vi "Configuration Tool Main.vi"() -> ()   [LabVIEW 2019, in "Configuration Tool.lvlib"]
doc: "This is the main VI for the configuration editor."
uses:
  Configuration Tool.lvlib
  Controls/StateCluster.ctl
  <vilib>/NI/Configuration Framework/Repository/NISE_CEF_Repository.lvclass
  <vilib>/NI/Configuration Framework/Node/NodeRef.ctl
  <vilib>/NI/Configuration Framework/Node/NISE_CEF_Node.lvclass
  <vilib>/NI/Configuration Framework/Node/StandardEvents.ctl
  <vilib>/NI/Configuration Framework/Node/UserEventRef.ctl
  <vilib>/NI/Configuration Framework/Controls/EventCluster.ctl
  <vilib>/NI/Configuration Framework/Node/NodeChangeEvent.ctl
  <vilib>/NI/Configuration Framework/Node/CacheState.ctl
  <vilib>/NI/Configuration Framework/Node/RefreshUIEvent.ctl
  <vilib>/NI/Configuration Framework/Node/StopEvent.ctl
  <vilib>/NI/Configuration Framework/glyph manager/glyph manager.ctl
  <vilib>/picture/picture.llb/imagedata.ctl
  Controls/AddMessage.ctl
  Controls/MoveMessage.ctl
  <vilib>/Utility/error.llb/DialogType.ctl
  Classes/CustomDeviceRepo/CustomDeviceRepo.lvclass
  C:/Program Files (x86)/National Instruments/LabVIEW 2019/vi.lib/NI/Configuration Framework/Repository/NISE_CEF_Repository.lvclass
  <vilib>/Utility/sysdir.llb/System Directory Type.ctl
  <vilib>/NI/AMC/Read Termination Message.vi
  <vilib>/NI/AMC/Create Single Message.vi
  <vilib>/NI/AMC/Update Message Routing Info.vi
  subVI/Global Settings.vi
  <vilib>/NI/AMC/Globals.vi
  <vilib>/NI/AMC/Send Message.vi
  <vilib>/NI/AMC/AMC.lvlib
  <vilib>/NI/Configuration Framework/NISE_CEF_TreeControl.lvlib
  <vilib>/NI/Configuration Framework/glyph manager/glyph manager.lvlib
panel:
  in  "Target Project":string(combo)
  in  "VeriStand Version":string(combo)
  in  "View":string(tree)
  in  "Exit":bool
  out "Status":string
  # "Custom Device XML Editor"
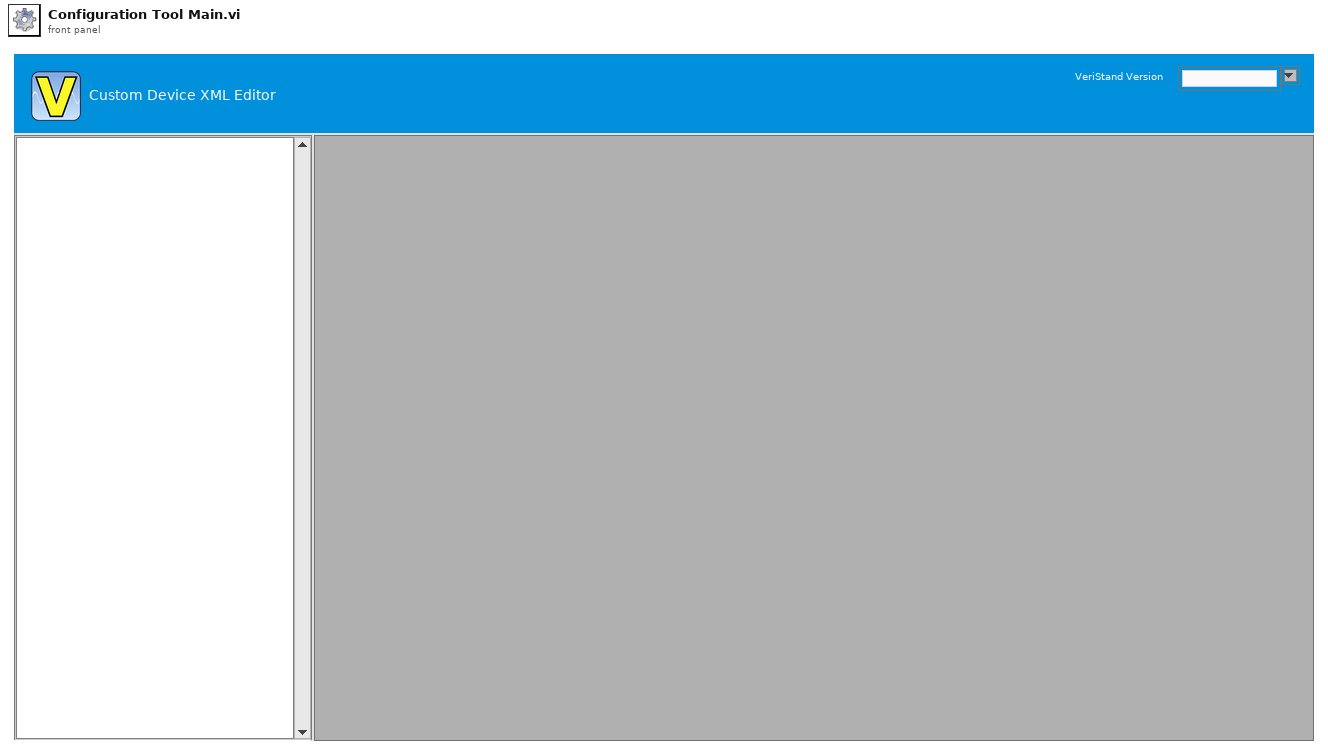
[diagram p1: front panel]
types:
  T1 = typedef "Configuration Tool.lvlib/StateCluster.ctl" = cluster{"repository":refnum<class "NISE_CEF_Repository.lvclass">, "root":T2, "unsaved changes":bool, "current path":path, "standard events":T3, "classes path":path, "glyph manager":T9}
  T2 = typedef "NISE_CEF_Node.lvclass/NodeRef.ctl" = refnum<data-value>
  T3 = typedef "NISE_CEF_Node.lvclass/StandardEvents.ctl" = cluster{"user event":T4, "node change":T5, "cache state":T6, "refresh UI":T7, "stop event":T8}
  T4 = typedef "NISE_CEF_Node.lvclass/UserEventRef.ctl" = refnum<user-event>
  T5 = typedef "NISE_CEF_Node.lvclass/NodeChangeEvent.ctl" = refnum<user-event>
  T6 = typedef "NISE_CEF_Node.lvclass/CacheState.ctl" = refnum<user-event>
  T7 = typedef "NISE_CEF_Node.lvclass/RefreshUIEvent.ctl" = refnum<user-event>
  T8 = typedef "NISE_CEF_Node.lvclass/StopEvent.ctl" = refnum<user-event>
  T9 = typedef "glyph manager.lvlib/glyph manager.ctl" = cluster{"search paths":path[], "glyph map":variant, "base glyphs":T10[], "desired overlays":string[]}
  T10 = typedef "imagedata.ctl" = cluster{"image type":i32, "image depth":i32, "image":u8[], "mask":u8[], "colors":u32[], "Rectangle":cluster{"left":i16, "top":i16, "right":i16, "bottom":i16}}
  T11 = cluster{"Names":string[], "Project refs":refnum<vi>[]}
  T12 = typedef "AMC.lvlib/Message Queue.ctl" = refnum<queue>
  T13 = typedef "Configuration Tool.lvlib/AddMessage.ctl" = cluster{"node type":string, "to add to":string}
  T14 = typedef "Configuration Tool.lvlib/MoveMessage.ctl" = cluster{"node ref":T2, "new parent":T2}
  T15 = typedef "Configuration Tool.lvlib/FilePaths.ctl" = cluster{"glyphs":path, "classes":path}
  T16 = typedef "DialogType.ctl" = u16
  T17 = typedef "System Directory Type.ctl" = i32
  T18 = typedef "NISE_CEF_Node.lvclass/Summary.ctl" = cluster{"ID":string, "parent ID":string, "node type":string, "text":string, "additional text":string, "glyph":string, "depth":i32, "glyph overlay":string}
  T19 = typedef "LVPoint32TypeDef.ctl" = cluster{"Horizontal":i32, "Vertical":i32}
  T20 = cluster{"data name":string, "drag data":variant}[]
  T21 = typedef "NISE_CEF_Node.lvclass/NodeMenuOptions.ctl" = cluster{"removable":bool, "movable":bool, "duplicate":bool}
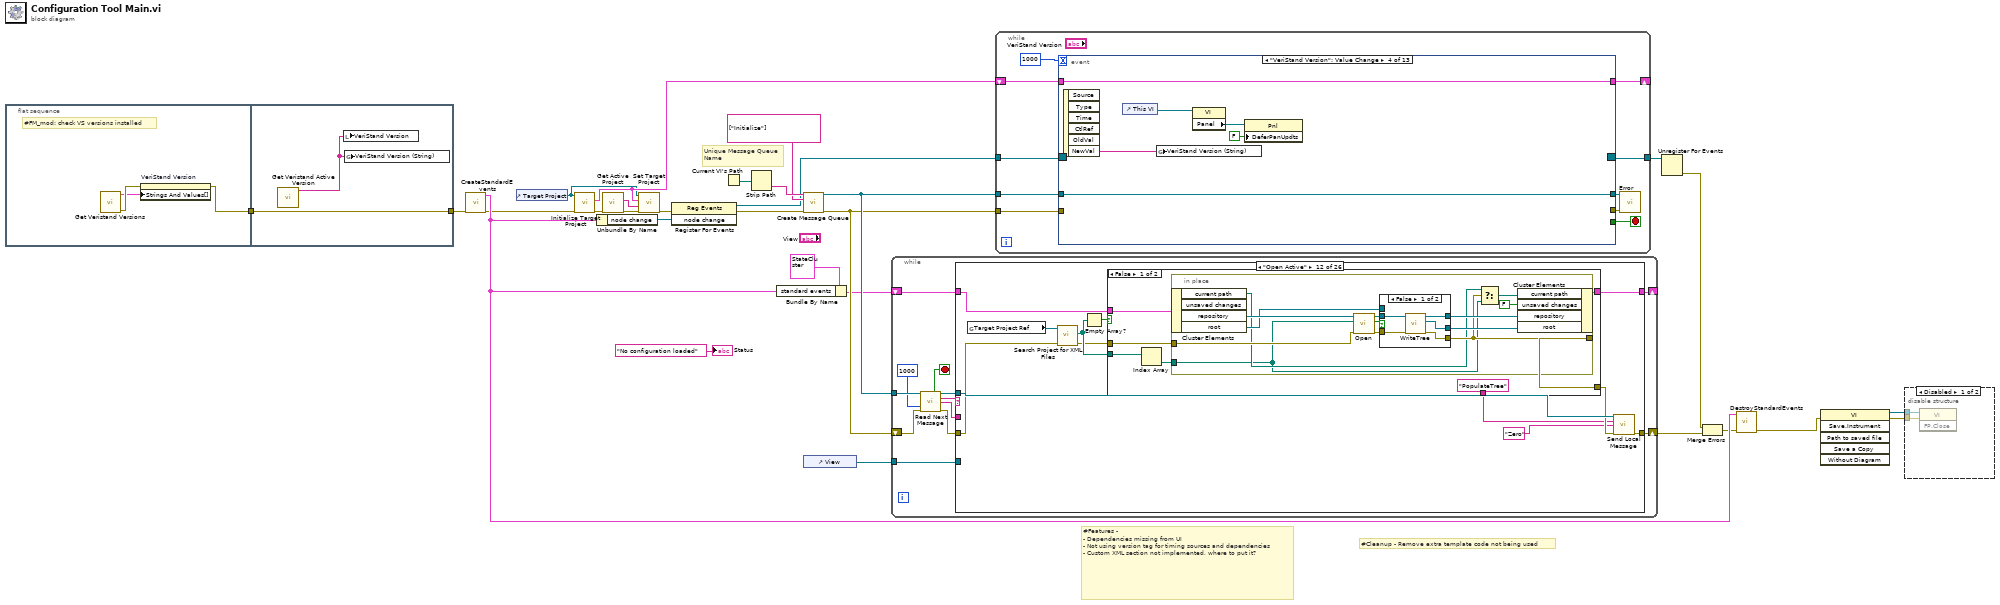
[diagram p0: block diagram]
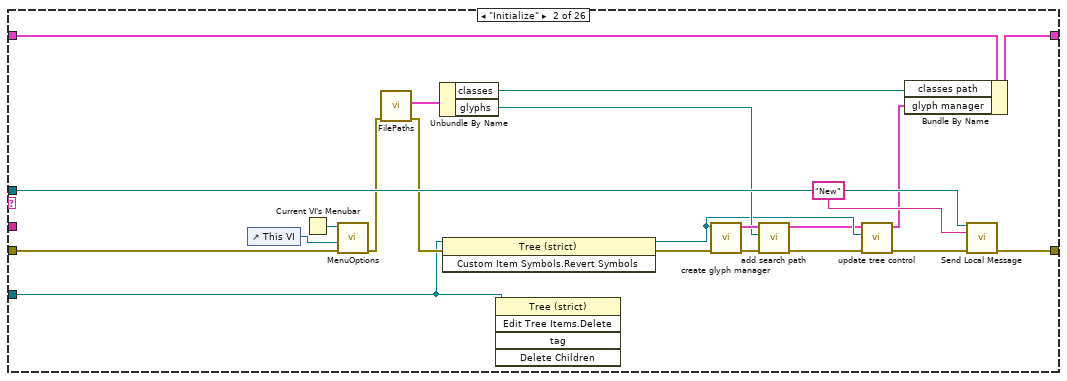
[diagram p4: hidden frame]
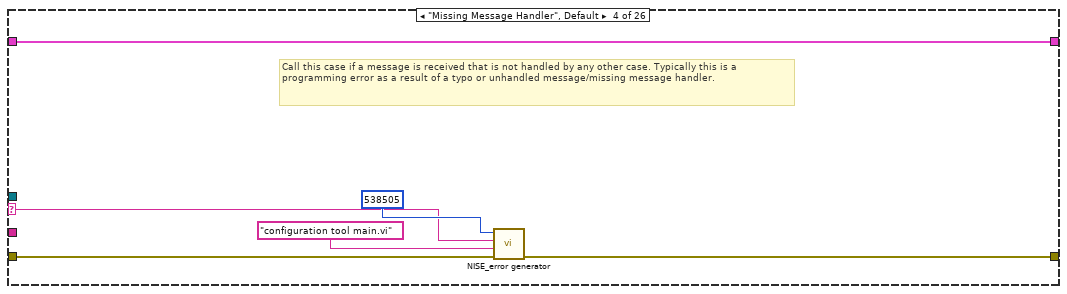
[diagram p6: hidden frame]
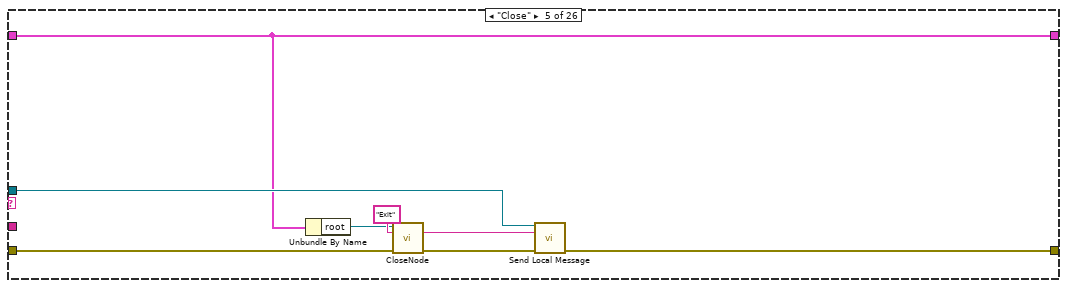
[diagram p7: hidden frame]
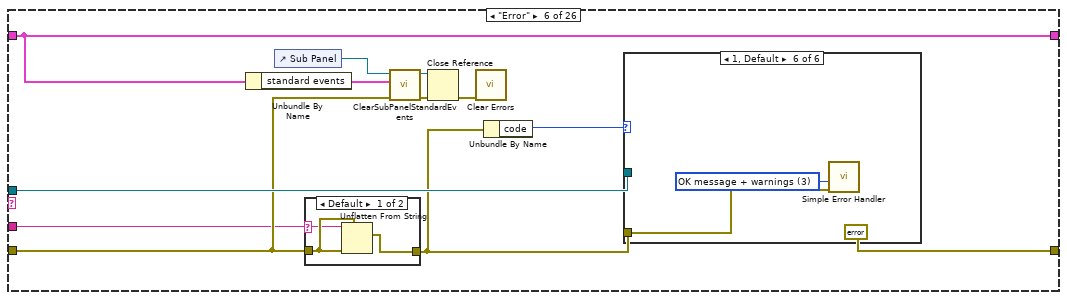
[diagram p8: hidden frame]
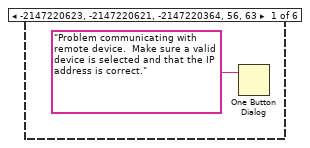
[diagram p10: hidden frame]
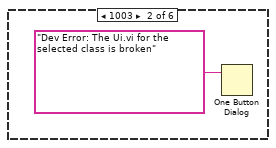
[diagram p11: hidden frame]
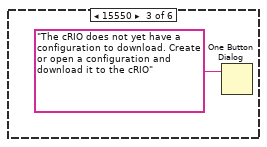
[diagram p12: hidden frame]
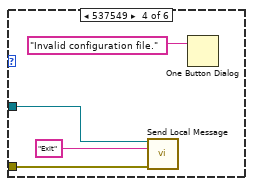
[diagram p13: hidden frame]
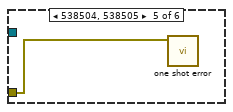
[diagram p14: hidden frame]
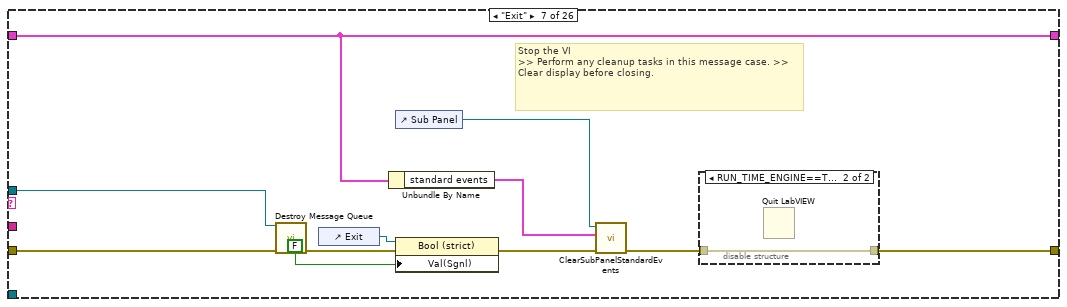
[diagram p15: hidden frame]
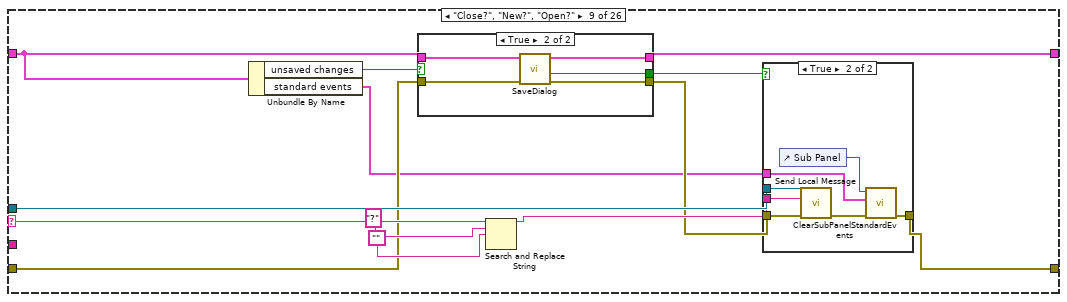
[diagram p18: hidden frame]
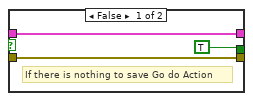
[diagram p19: hidden frame]
diagram:
  # "#Cleanup - Remove extra template code not being used"
  # "#Features - \n- Dependencies missing from UI\n- Not using version tag for timing sources and dependencies\n- Custom XML section not implemented, where to put it?"
  # "Unique Message Queue Name"
  n1 = flat-sequence {
    tunnel: [w31] -> w1
    tunnel: [w34] -> w2
    tunnel: w1 -> [w34]
    frame #0 {
      # "#FM_mod: check VS versions installed"
      n2 = call "Get Veristand Versions.vi"() -> ("error out"=w32:errorcluster, "Versions"=w30:cluster{"String":string, "Value":string}[])  [unwired: 10 in]
      n3 = property on="VeriStand Version" class="CmbBox"(error in=w32, "Strings And Values[]"=w30) -> (error out=w31:errorcluster)  [unwired: 1 in, 1 out]
    }
    frame #1 {
      n4 = call "Get Veristand Active Version.vi"() -> ("Version"=w33:string)  [unwired: 11 in]
      n5 = local write "VeriStand Version"(w33) -> ()
      n6 = global write "Global Settings.vi" "VeriStand Version (String)"(w33) -> ()
    }
  }
  n7 = call <vilib>:"CreateStandardEvents.vi"("error in"=w2) -> ("error out"=w8:errorcluster, "standard events"=w19:T3)  [unwired: 9 in]
  n8 = control-ref of="Target Project"() -> (w9:refnum<vi>)
  n9 = call "Initialize Target Project.vi"("error in (no error)"=w8, "ComboBox in"=w9) -> ("error out"=w13:errorcluster, "Projects"=w11:T11)  [unwired: 8 in]
  n10 = Unbundle By Name(w19) -> ("node change"=w24:T5)
  n11 = call "Get Active Project.vi"("error in (no error)"=w13) -> ("error out"=w12:errorcluster, "Name"=w10:string)  [unwired: 7 in, 2 out]
  n12 = call "Set Target Project.vi"("error in (no error)"=w12, "Target Project"=w10, "Projects"=w11, "ComboBox Ref"=w9) -> ("error out"=w7:errorcluster)  [unwired: 7 in]
  n13 = register-events(error in=w7, w24) -> (reference out=w18:refnum<event-registration>, error out=w23:errorcluster)  [unwired: 1 in]
  n14 = Current VI's Path() -> (path=w28:path)
  n15 = Strip Path(path=w28) -> (name=w29:string)  [unwired: 1 out]
  n16 = Bundle By Name(cluster=T1 {"repository"=refnum, "root"=refnum, "unsaved changes"=FALSE, "current path"=path "", "standard events"={"user event"=refnum, "node change"=refnum, "cache state"=refnum, "refresh UI"=refnum, "stop event"=refnum}, "classes path"=path "", "glyph manager"={"search paths"=[], "glyph map"=variant, "base glyphs"=[], "desired overlays"=[]}}, "standard events"=w19) -> (w21:T1)
  n17 = call <vilib>:"Create Message Queue.vi"("message queue name"=w29, "initial message names"=string[] ["Initialize"], "error in"=w23) -> ("message queue out"=w26:T12, "error out"=w25:errorcluster)  [unwired: 11 in]
  n18 = control-ref of="View"() -> (w17:refnum<vi>)
  n19 = while "Message Processor" {
    shift-right: [w42] -> w20
    shift-left: w25 -> [w41]
    tunnel: w26 -> [w40]
    shift-right: [w38] -> _
    shift-left: w21 -> [w37]
    tunnel: w17 -> [w35]
    stop <- w46 stop-if-true
    n20 = call <vilib>:"Read Next Message.vi"("message queue in"=w40, "timeout (1 ms)"=1000, "error in"=w41) -> ("exit process?"=w46:bool, "message queue out"=w36:T12, "message name"=w45:string, "message value"=w44:string, "error out"=w43:errorcluster)  [unwired: 5 in, 3 out]
    n21 = case shown="\"Open Active\"" w45 {
      selector: w45 -> [_ _ _ w74 _ _ _ _ w135 _ _ _ _ _ _ _ _ _ w393 _ _ _ _ _ _ _]
      tunnel: w44 -> [_ _ _ _ _ w87 _ _ _ _ _ _ _ _ w302 _ w354 w371 w391 w443 w467 w479 _ w528 w548 w555]
      tunnel: w43 -> [w48 w70 w72 w77 w80 w90 w122 w126 w128 w166 w185 w228 w272 w294 w309 w322 w347 w370 w396 w445 w466 w496 w518 w527 w546 w556]
      tunnel: [w48 w66 w72 w75 w84 errorcluster {"status"=FALSE, "code"=0, "source"=""} ("error out") w114 w126 w139 w172 w181 w233 w269 w296 w306 w322 w326 w374 w399 w447 w463 w483 w514 w524 w541 w554] -> w42
      tunnel: [w47 w62 w71 w78 w82 w94 w113 w125 w130 w170 w186 w236 w275 w295 w303 w321 w342 w367 w400 w446 w468 w489 w517 w522 w549 w551] -> w38
      tunnel: w37 -> [w47 w63 w71 w78 w82 w94 w113 w125 w131 w168 w187 w237 w274 w293 w304 w321 w345 w368 w400 w438 w468 w498 w517 w522 w549 w557]
      tunnel: w36 -> [_ w65 _ _ w83 w97 w121 _ w138 w171 w183 w235 _ _ w305 _ w323 _ w394 _ _ _ _ w523 w540 w553]
      tunnel: w35 -> [_ w49 _ _ _ _ _ _ _ _ _ _ _ _ _ _ w343 w363 w388 w440 w461 w485 _ _ _ _]
      frame "------------Generic Operations------------" {
        # "Dummy case to add a seperation in the Case Structure menu"
      }
      frame "Initialize" {
        n22 = control-ref of="This VI"() -> (w69:refnum<vi>)
        n23 = Current VI's Menubar() -> (w68:refnum<k9>)
        n24 = call "MenuOptions.vi"("error in"=w70, "VI ref"=w69, "menu ref in"=w68) -> ("error out"=w61:errorcluster)  [unwired: 7 in, 1 out]
        n25 = call "FilePaths.vi"("error in"=w61) -> ("error out"=w54:errorcluster, "paths"=w64:T15)  [unwired: 9 in]
        n26 = Unbundle By Name(w64) -> ("classes"=w60:path, "glyphs"=w56:path)
        n27 = invoke class="Tree (strict)" method="Custom Item Symbols.Revert Symbols"(reference=w49, error in=w54) -> (reference out=w52:refnum<vi>, error out=w53:errorcluster)  [unwired: 1 in, 1 out]
        n28 = invoke class="Tree (strict)" method="Edit Tree Items.Delete"(reference=w49) -> ()  [unwired: 4 in, 5 out]
        n29 = call <vilib>:"create glyph manager.vi"("error in"=w53, "tree ref (for default symbols)"=w52) -> ("error out"=w59:errorcluster, "glyph manager"=w58:T9)  [unwired: 8 in]
        n30 = call <vilib>:"add search path.vi"("error in"=w59, "search path"=w56, "glyph manager in"=w58) -> ("error out"=w51:errorcluster, "glyph manager out"=w50:T9)  [unwired: 7 in]
        n31 = call <vilib>:"update tree control.vi"("error in"=w51, "tree reference"=w52, "glyph manager in"=w50) -> ("error out"=w57:errorcluster, "glyph manager out"=w55:T9)  [unwired: 7 in]
        n32 = Bundle By Name(cluster=w63, "classes path"=w60, "glyph manager"=w55) -> (w62:T1)
        n33 = call <vilib>:"Send Local Message.vi"("message queue in"=w65, "message name"="New" ("Message Name"), "error in"=w57) -> ("error out"=w66:errorcluster)  [unwired: 10 in, 2 out]
      }
      frame "", "Idle" {
      }
      frame "Missing Message Handler", Default {
        # "Call this case if a message is received that is not handled by any other case. Typically this is a programming error as a result of a typo or unhandled message/missing message handler."
        n34 = call <vilib>:"NISE_error generator.vi"("error in"=w77, "source"="configuration tool main.vi", "append error message"=w74, "error code (0)"=538505) -> ("error out"=w75:errorcluster)  [unwired: 5 in]
      }
      frame "Close" {
        n35 = Unbundle By Name(w82) -> ("root"=w81:T2)
        n36 = call <vilib>:"CloseNode.vi"("error in"=w80, "node ref"=w81) -> ("error out"=w79:errorcluster)  [unwired: 9 in]
        n37 = call <vilib>:"Send Local Message.vi"("message queue in"=w83, "message name"="Exit", "error in"=w79) -> ("error out"=w84:errorcluster)  [unwired: 10 in, 2 out]
      }
      frame "Error" {
        n38 = Unbundle By Name(w94) -> ("standard events"=w86:T3)
        n39 = control-ref of="Sub Panel"() -> (w93:refnum<vi>)
        n40 = case shown="Default" w87 {
          selector: w87 -> [w99 _]
          tunnel: w90 -> [w100 w101]
          tunnel: [w98 w101] -> w89
          frame Default {
            n41 = Unflatten From String(type=w100, binary string=w99, error in (no error)=w100) -> (value=w98:errorcluster)  [unwired: 2 in, 2 out]
          }
          frame "" {
          }
        }
        n42 = call <vilib>:"ClearSubPanelStandardEvents.vi"("error in"=w90, "standard events"=w86, "sub panel ref in"=w93) -> ("error out"=w92:errorcluster, "sub panel ref out"=w91:refnum<vi>)  [unwired: 7 in]
        n43 = Close Reference(reference=w91, error in (no error)=w92) -> (error out=w88:errorcluster)
        n44 = call <vilib>:"Clear Errors.vi"("error in (no error)"=w88) -> ()  [unwired: 5 in, 2 out]
        n45 = Unbundle By Name(w89) -> ("code"=w95:i32)
        n46 = case shown="1, Default" w95 {
          tunnel: w97 -> [_ _ _ w107 _ _]
          tunnel: w89 -> [_ _ _ w106 w109 w111]
          frame -2147220623, -2147220621, -2147220364, 56, 63 {
            n47 = One Button Dialog(message="Problem communicating with remote device.  Make sure a valid device is selected and that the IP address is correct.") -> ()  [unwired: 1 in, 1 out]
          }
          frame 1003 {
            n48 = One Button Dialog(message="Dev Error: The Ui.vi for the selected class is broken") -> ()  [unwired: 1 in, 1 out]
          }
          frame 15550 {
            n49 = One Button Dialog(message="The cRIO does not yet have a configuration to download. Create or open a configuration and download it to the cRIO") -> ()  [unwired: 1 in, 1 out]
          }
          frame 537549 {
            n50 = call <vilib>:"Send Local Message.vi"("message queue in"=w107, "message name"="Exit", "error in"=w106) -> ()  [unwired: 10 in, 3 out]
            n51 = One Button Dialog(message="Invalid configuration file.") -> ()  [unwired: 1 in, 1 out]
          }
          frame 538504, 538505 {
            n52 = call <vilib>:"one shot error.vi"("error in"=w109) -> ()  [unwired: 11 in]
          }
          frame 1, Default {
            w110 = T16 3 items=["no dialog", "OK message", "continue or stop message", "OK message + warnings", "continue/stop + warnings"] ("type of dialog (OK msg:1)")
            n53 = call <vilib>:"Simple Error Handler.vi"("type of dialog (OK msg:1)"=w110, "error in (no error)"=w111) -> ()  [unwired: 8 out]
          }
        }
      }
      frame "Exit" {
        # "Stop the VI                                                                             >> Perform any cleanup tasks in this message case. >> Clear display before closing."
        n54 = call <vilib>:"Destroy Message Queue.vi"("message queue in"=w121, "error in"=w122) -> ("error out"=w118:errorcluster)  [unwired: 11 in, 2 out]
        n55 = control-ref of="Exit"() -> (w120:refnum<vi>)
        n56 = Unbundle By Name(w113) -> ("standard events"=w112:T3)
        n57 = control-ref of="Sub Panel"() -> (w117:refnum<vi>)
        n58 = property class="Bool (strict)"(reference=w120, error in=w118, "Val(Sgnl)"=FALSE ("Exit")) -> (error out=w116:errorcluster)  [unwired: 1 out]
        n59 = call <vilib>:"ClearSubPanelStandardEvents.vi"("error in"=w116, "standard events"=w112, "sub panel ref in"=w117) -> ("error out"=w115:errorcluster)  [unwired: 7 in, 1 out]
        n60 = disable-structure shown="RUN_TIME_ENGINE==True" {
          disable-tunnel: [w123 w124] -> w114
          disable-tunnel: w115 -> [w123 w124]
          frame condition #0 (active) {
          }
          frame condition #1 {
            n61 = Quit LabVIEW() -> ()  [unwired: 1 in]
          }
        }
      }
      frame "------------Menu Operations--------------" {
        # "Dummy case to add a seperation in the Case Structure menu"
      }
      frame "Close?", "New?", "Open?" {
        n62 = Unbundle By Name(w131) -> ("unsaved changes"=w133:bool, "standard events"=w127:T3)
        n63 = case shown="True" w133 {
          tunnel: [TRUE ("SaveFlag") w147] -> w132
          tunnel: w131 -> [w141 w146]
          tunnel: [w141 w145] -> w130
          tunnel: w128 -> [w140 w144]
          tunnel: [w140 w143] -> w129
          frame False {
            # "If there is nothing to save Go do Action"
          }
          frame True {
            n64 = call "SaveDialog.vi"("error in"=w144, "state in"=w146) -> ("error out"=w143:errorcluster, "new"=w147:bool, "state out"=w145:T1)  [unwired: 7 in]
          }
        }
        n65 = Search and Replace String(input string=w135, search string="?", replace string="") -> (result string=w134:string)  [unwired: 5 in, 3 out]
        n66 = case shown="True" w132 {
          tunnel: w129 -> [w148 w155]
          tunnel: [w148 w151] -> w139
          tunnel: w138 -> [_ w154]
          tunnel: w134 -> [_ w153]
          tunnel: w127 -> [_ w149]
          frame False {
          }
          frame True {
            n67 = control-ref of="Sub Panel"() -> (w150:refnum<vi>)
            n68 = call <vilib>:"Send Local Message.vi"("message queue in"=w154, "message name"=w153, "error in"=w155) -> ("error out"=w152:errorcluster)  [unwired: 10 in, 2 out]
            n69 = call <vilib>:"ClearSubPanelStandardEvents.vi"("error in"=w152, "standard events"=w149, "sub panel ref in"=w150) -> ("error out"=w151:errorcluster)  [unwired: 7 in, 1 out]
          }
        }
      }
      frame "New" {
        # "#Change - Won't allow creating so changing unsaved constant to F"
        n70 = Unbundle By Name(w168) -> ("classes path"=w167:path)
        n71 = Current VI's Menubar() -> (w162:refnum<k9>)
        n72 = call-dynamic "Initialize.vi"("error in"=w166, "path"=w167, "repository in"=refnum<class "CustomDeviceRepo.lvclass"> refnum ("CustomDeviceRepo.lvclass")) -> ("error out"=w165:errorcluster, "repository out"=w164:refnum<class "CustomDeviceRepo.lvclass">)  [unwired: 7 in]
        n73 = call-dynamic "GenerateMenu.vi"("error in"=w165, "menu ref in"=w162, "NISE_CEF_Repository in"=w164) -> ("error out"=w161:errorcluster, "NISE_CEF_Repository out"=w163:refnum<class "CustomDeviceRepo.lvclass">)  [unwired: 6 in, 1 out]
        n74 = call "Get Active Project.vi"() -> ("No Active Project?"=w159:bool)  [unwired: 8 in, 3 out]
        n75 = Bundle By Name(cluster=w168, "unsaved changes"=FALSE ("SaveFlag"), "repository"=w163) -> (w170:T1)
        n76 = Select(t="Idle", s=w159, f="Open Active") -> (s? t:f=w156:string)
        n77 = call <vilib>:"Send Local Message.vi"("message queue in"=w171, "message name"=w156, "error in"=w161) -> ("error out"=w172:errorcluster)  [unwired: 10 in, 2 out]
      }
      frame "Open" {
        w180 = T17 6 items=["User Home"=0, "User Desktop"=1, "User Documents"=2, "User Application Data"=3, "User Preferences"=4, "User Temporary"=5, "Public Documents"=6, "Public Application Data"=7, "Public Preferences"=8, "Public Cache"=13, "System Core Libraries"=9, "System Installed Libraries"=10, "Application Files"=11, "Boot Volume Root"=12] ("system directory type")
        n78 = disable-structure shown="Disabled" {
          disable-tunnel: [w188 w190] -> w173
          frame Disabled {
            n79 = global read "Global Settings.vi" "VeriStand Version"() -> (w189:enum16{"2013", "2014", "2015", "2016"})
            n80 = Format Into String(w189) -> (resulting string=w188:string)  [unwired: 3 in, 1 out]
          }
          frame Enabled {
            # "#FM_mod: using string instead"
            n81 = global read "Global Settings.vi" "VeriStand Version (String)"() -> (w190:string)
          }
        }
        n82 = Search and Replace String(input string="National Instruments\\NI VeriStand XXXX\\Custom Devices", search string="XXXX", replace string=w173) -> (result string=w176:string)  [unwired: 5 in, 3 out]
        n83 = call <vilib>:"Get System Directory.vi"("system directory type"=w180) -> ("system directory"=w177:path)  [unwired: 10 in]
        n84 = Build Path(base path=w177, name or relative path=w176) -> (appended path=w175:path)
        n85 = in-place {
          in-place-border: w185 -> [w196]
          in-place-border: [w195] -> w182
          in-place-border: w175 -> [w191]
          n86 = in-place-cluster #1(w187) -> ("current path"=w193:path, "repository"=w204:refnum<class "NISE_CEF_Repository.lvclass">, "root"=w200:T2)  [unwired: 1 out]
          n87 = call "FileDialog.vi"("error in"=w196, "start path"=w191) -> ("error out"=w197:errorcluster, "cancelled"=w198:bool, "selected path"=w194:path)  [unwired: 7 in]
          n88 = Compound Arithmetic op=OR(invert w198) -> (w199:bool)
          n89 = case shown="True" w199 {
            tunnel: w204 -> [w205 w217]
            tunnel: [w205 w215] -> w202
            tunnel: [w206 w213] -> w195
            tunnel: [w207 w212] -> w201
            tunnel: w194 -> [_ w210]
            tunnel: w197 -> [w206 w209]
            tunnel: w200 -> [w207 w208]
            frame False {
            }
            frame True {
              n90 = call-dynamic "Open.vi"("error in"=w209, "file path"=w210, "repository in"=w217) -> ("error out"=w214:errorcluster, "invalid?"=w211:bool, "repository out"=w216:refnum<class "NISE_CEF_Repository.lvclass">)  [unwired: 6 in]
              n91 = case shown="False" w211 {
                tunnel: w216 -> [w222 w225]
                tunnel: [w221 w225] -> w215
                tunnel: w214 -> [w220 w224]
                tunnel: [w219 w224] -> w213
                tunnel: [w218 w223] -> w212
                tunnel: w208 -> [_ w223]
                frame False {
                  n92 = call-dynamic "WriteTree.vi"("error in"=w220, "repository in"=w222) -> ("error out"=w219:errorcluster, "root"=w218:T2, "repository out"=w221:refnum<class "NISE_CEF_Repository.lvclass">)  [unwired: 7 in]
                }
                frame True {
                }
              }
            }
          }
          n93 = Select(t=w193, s=w195, f=w194) -> (s? t:f=w192:path)
          n94 = in-place-cluster #1("current path"=w192, "unsaved changes"=FALSE ("SaveFlag"), "repository"=w202, "root"=w201) -> (w186:T1)
        }
        n95 = call <vilib>:"Send Local Message.vi"("message queue in"=w183, "message name"="PopulateTree", "message value"="Zero", "error in"=w182) -> ("error out"=w181:errorcluster)  [unwired: 9 in, 2 out]
      }
      frame "Open Active" {
        n96 = global read "Global Settings.vi" "Target Project Ref"() -> (w231:refnum<vi>)
        n97 = call "Search Project for XML Files.vi"("error in (no error)"=w228, "project reference"=w231) -> ("error out"=w227:errorcluster, "xml files found"=w230:path[])  [unwired: 8 in]
        n98 = Empty Array?(array=w230) -> (empty?=w229:bool)
        n99 = case shown="False" w229 {
          tunnel: w237 -> [w244 w268]
          tunnel: [w243 w268] -> w236
          tunnel: w227 -> [w242 w267]
          tunnel: [w241 w267] -> w234
          tunnel: w230 -> [w239 _]
          tunnel: ["PopulateTree" "Idle"] -> w226
          frame False {
            n100 = Index Array(array=w239) -> (element=w240:path)  [unwired: 1 in]
            n101 = in-place {
              in-place-border: w242 -> [w252]
              in-place-border: [w251] -> w241
              in-place-border: w240 -> [w245]
              n102 = in-place-cluster #2(w244) -> ("current path"=w250:path, "repository"=w257:refnum<class "NISE_CEF_Repository.lvclass">, "root"=w253:T2)  [unwired: 1 out]
              n103 = call-dynamic "Open.vi"("error in"=w252, "file path"=w245, "repository in"=w257) -> ("error out"=w247:errorcluster, "invalid?"=w246:bool, "repository out"=w248:refnum<class "NISE_CEF_Repository.lvclass">)  [unwired: 6 in]
              n104 = case shown="False" w246 {
                tunnel: w248 -> [w262 w265]
                tunnel: [w261 w265] -> w255
                tunnel: w247 -> [w260 w264]
                tunnel: [w259 w264] -> w251
                tunnel: [w258 w263] -> w254
                tunnel: w253 -> [_ w263]
                frame False {
                  n105 = call-dynamic "WriteTree.vi"("error in"=w260, "repository in"=w262) -> ("error out"=w259:errorcluster, "root"=w258:T2, "repository out"=w261:refnum<class "NISE_CEF_Repository.lvclass">)  [unwired: 7 in]
                }
                frame True {
                }
              }
              n106 = Select(t=w250, s=w251, f=w245) -> (s? t:f=w249:path)
              n107 = in-place-cluster #2("current path"=w249, "unsaved changes"=FALSE ("SaveFlag"), "repository"=w255, "root"=w254) -> (w243:T1)
            }
          }
          frame True {
          }
        }
        n108 = call <vilib>:"Send Local Message.vi"("message queue in"=w235, "message name"=w226, "message value"="Zero", "error in"=w234) -> ("error out"=w233:errorcluster)  [unwired: 9 in, 2 out]
      }
      frame "Save" {
        n109 = in-place {
          in-place-border: w272 -> [w279]
          in-place-border: [w278] -> w271
          in-place-border: [w276] -> w270
          n110 = in-place-cluster #3(w274) -> ("current path"=w277:path, "root"=w280:T2, "repository"=w282:refnum<class "NISE_CEF_Repository.lvclass">)
          n111 = Empty String/Path?(string/path=w277) -> (empty?=w276:bool)
          n112 = call-dynamic "ReadTree.vi"("error in"=w279, "root"=w280, "repository in"=w282) -> ("error out"=w278:errorcluster, "repository out"=w281:refnum<class "NISE_CEF_Repository.lvclass">)  [unwired: 7 in]
          n113 = in-place-cluster #3("current path"=w277, "root"=w280, "repository"=w281) -> (w273:T1)
        }
        n114 = case shown="False" w270 {
          tunnel: w273 -> [w286 w288]
          tunnel: [w285 w287] -> w275
          tunnel: [w284 w289] -> w269
          tunnel: w271 -> [w283 w290]
          frame False {
            n115 = call "Save.vi"("error in"=w283, "state in"=w286) -> ("error out"=w284:errorcluster, "state out"=w285:T1)  [unwired: 8 in]
          }
          frame True {
            # "Empty path use Dialog"
            n116 = call "SaveAs.vi"("error in"=w290, "state in"=w288) -> ("error out"=w289:errorcluster, "state out"=w287:T1)  [unwired: 7 in, 1 out]
          }
        }
      }
      frame "SaveAs" {
        n117 = in-place {
          in-place-border: w294 -> [w298]
          in-place-border: [w297] -> w292
          n118 = in-place-cluster #4(w293) -> ("root"=w299:T2, "repository"=w301:refnum<class "NISE_CEF_Repository.lvclass">)
          n119 = call-dynamic "ReadTree.vi"("error in"=w298, "root"=w299, "repository in"=w301) -> ("error out"=w297:errorcluster, "repository out"=w300:refnum<class "NISE_CEF_Repository.lvclass">)  [unwired: 7 in]
          n120 = in-place-cluster #4("root"=w299, "repository"=w300) -> (w291:T1)
        }
        n121 = call "SaveAs.vi"("error in"=w292, "state in"=w291) -> ("error out"=w296:errorcluster, "state out"=w295:T1)  [unwired: 7 in, 1 out]
      }
      frame "Custom View" {
        n122 = in-place {
          in-place-border: w309 -> [w320]
          in-place-border: [w319] -> w307
          in-place-border: w302 -> [w310]
          n123 = in-place-cluster #5(w304) -> ("repository"=w314:refnum<class "NISE_CEF_Repository.lvclass">, "root"=w313:T2)
          n124 = call-dynamic "ReadTree.vi"("error in"=w320, "root"=w313, "repository in"=w314) -> ("error out"=w317:errorcluster, "repository out"=w316:refnum<class "NISE_CEF_Repository.lvclass">)  [unwired: 7 in]
          n125 = call-dynamic "CustomView.vi"("error in"=w317, "view name"=w310, "repository in"=w316) -> ("error out"=w318:errorcluster, "repository out"=w315:refnum<class "NISE_CEF_Repository.lvclass">)  [unwired: 7 in]
          n126 = call-dynamic "WriteTree.vi"("error in"=w318, "repository in"=w315) -> ("error out"=w319:errorcluster, "root"=w311:T2, "repository out"=w312:refnum<class "NISE_CEF_Repository.lvclass">)  [unwired: 7 in]
          n127 = in-place-cluster #5("repository"=w312, "root"=w311) -> (w303:T1)
        }
        n128 = call <vilib>:"Send Local Message.vi"("message queue in"=w305, "message name"="PopulateTree", "error in"=w307) -> ("error out"=w306:errorcluster)  [unwired: 10 in, 2 out]
      }
      frame "-------TreeControl Operations-----------" {
        # "Dummy case to add a seperation in the Case Structure menu"
      }
      frame "AddNode" {
        # "#Change - Added ability for added nodes\nto then add children"
        # "#Change - Had to make own copy\nof add node since CEF framework\ndoesn't let you pass params to init"
        # "#Change - Look for potential\ndashes for menu items with\nparameterized options"
        n129 = Unflatten From String(type=T13 {"node type"="", "to add to"=""} ("input cluster"), binary string=w354) -> (value=w352:T13)  [unwired: 3 in, 2 out]
        n130 = Unbundle By Name(w352) -> ("to add to"=w350:string, "node type"=w332:string)
        n131 = Match Pattern(string=w332, regular expression="\\-") -> (before substring=w331:string, after substring=w330:string)  [unwired: 1 in, 2 out]
        n132 = in-place {
          in-place-border: w347 -> [w360]
          in-place-border: [w359] -> w346
          in-place-border: w331 -> [w358]
          in-place-border: [w357] -> w344
          n133 = in-place-cluster #6(w345) -> ("repository"=w362:refnum<class "NISE_CEF_Repository.lvclass">)
          n134 = call-dynamic "GetClassPath.vi"("error in"=w360, "class name"=w358, "Repository in"=w362) -> ("error out"=w359:errorcluster, "class path"=w357:path, "Repository out"=w361:refnum<class "NISE_CEF_Repository.lvclass">)  [unwired: 6 in]
          n135 = in-place-cluster #6("repository"=w361) -> (w339:T1)
        }
        n136 = Unbundle By Name(w339) -> ("glyph manager"=w338:T9)
        n137 = call <vilib>:"Get LV Class Default Value.vi"("error in (no error)"=w346, "class path"=w344) -> ("error out"=w355:errorcluster, "object"=w356:refnum<class>)  [unwired: 8 in]
        n138 = To More Specific Class(target class=refnum<class "NISE_CEF_Node.lvclass"> refnum ("Node.lvclass"), reference=w356, error in=w355) -> (specific class reference=w340:refnum<class "NISE_CEF_Node.lvclass">, error out=w341:errorcluster)
        n139 = call-dynamic "AddGlyphtoGManager.vi"("error in"=w341, "glyph manager"=w338, "NISE_CEF_Node in"=w340) -> ("error out"=w336:errorcluster, "glyph manager out"=w337:T9, "NISE_CEF_Node out"=w335:refnum<class "NISE_CEF_Node.lvclass">)  [unwired: 6 in]
        n140 = Match Pattern(string=w330, regular expression="\\-") -> (before substring=w328:string, after substring=w325:string)  [unwired: 1 in, 2 out]
        n141 = call "Modified Framework AddNode.vi"("parameters"=w328, "error in"=w336, "node in"=w335, "parent node ID"=w350) -> ("error out"=w349:errorcluster, "summary"=w348:T18[], "ID of Added Node"=w324:string)  [unwired: 5 in]
        n142 = call <vilib>:"PopulateTreeSumaryWithGlyphManager.vi"("error in"=w349, "glyph manager"=w337, "summary"=w348, "tree ref in"=w343) -> ("error out"=w327:errorcluster, "glyph manager out"=w334:T9)  [unwired: 6 in]
        n143 = Bundle By Name(cluster=w339, "glyph manager"=w334) -> (w342:T1)
        n144 = call "Send Message to Create Child Object.vi"("Error In"=w327, "ID of Node to Add To"=w324, "node type"=w325, "Queue in"=w323) -> ("Error Out"=w326:errorcluster)  [unwired: 6 in, 1 out]
      }
      frame "Duplicate" {
        n145 = call <vilib>:"IDtoNode.vi"("error in"=w370, "ID"=w371) -> ("error out"=w372:errorcluster, "invalid Id"=w369:bool, "node ref"=w373:T2)  [unwired: 7 in]
        n146 = Unbundle By Name(w368) -> ("glyph manager"=w365:T9)
        n147 = case shown="False" w369 {
          tunnel: [w385 w387] -> w374
          tunnel: w373 -> [w384 _]
          tunnel: w372 -> [w381 w387]
          tunnel: w365 -> [w377 w386]
          tunnel: [w376 w386] -> w364
          tunnel: w363 -> [w375 _]
          frame False {
            n148 = call <vilib>:"DuplicateNode.vi"("same parent?"=TRUE ("s"), "error in"=w381, "node ref in"=w384) -> ("error out"=w382:errorcluster, "new node ref"=w383:T2)  [unwired: 7 in]
            n149 = call <vilib>:"Summary.vi"("error in"=w382, "node self ref"=w383) -> ("error out"=w379:errorcluster, "summary"=w378:T18[])  [unwired: 8 in]
            n150 = call <vilib>:"PopulateTreeSumaryWithGlyphManager.vi"("error in"=w379, "glyph manager"=w377, "summary"=w378, "tree ref in"=w375) -> ("error out"=w385:errorcluster, "glyph manager out"=w376:T9)  [unwired: 6 in]
          }
          frame True {
          }
        }
        n151 = Bundle By Name(cluster=w368, "unsaved changes"=TRUE, "glyph manager"=w364) -> (w367:T1)
      }
      frame "CustomMenuAction" {
        n152 = Match Pattern(string=w391, regular expression=":") -> (before substring=w390:string, after substring=w389:string)  [unwired: 1 in, 2 out]
        n153 = call <vilib>:"IDtoNode.vi"("error in"=w396, "ID"=w389) -> ("error out"=w397:errorcluster, "invalid Id"=w395:bool, "node ref"=w398:T2)  [unwired: 7 in]
        n154 = case shown="False" w395 {
          tunnel: [w406 w436] -> w399
          tunnel: w398 -> [w403 _]
          tunnel: w397 -> [w409 w436]
          tunnel: w394 -> [w410 _]
          tunnel: w393 -> [_ _]
          tunnel: w390 -> [w407 _]
          tunnel: w388 -> [w404 _]
          frame False {
            n155 = in-place {
              in-place-border: w410 -> [w434]
              in-place-border: w409 -> [w432]
              in-place-border: [w431] -> w405
              in-place-border: [w430] -> w408
              in-place-border: w407 -> [w429]
              in-place-border: w404 -> [w428]
              in-place-border: [w427] -> w402
              n156 = in-place-dvr #7(w403) -> (w435:refnum<class "NISE_CEF_Node.lvclass">)  [unwired: 1 out]
              n157 = call-dynamic "MenuHandler.vi"("tree control"=w428, "main message queue"=w434, "error in"=w432, "menu string"=w429, "NISE_CEF_Node in"=w435) -> ("error out"=w431:errorcluster, "refresh tree?"=w427:bool, "Unhandled"=w430:bool, "NISE_CEF_Node out"=w433:refnum<class "NISE_CEF_Node.lvclass">)  [unwired: 3 in]
              n158 = in-place-dvr #7(w433) -> (w401:T2)  [unwired: 1 out]
            }
            n159 = case shown="True" w408 {
              tunnel: w407 -> [_ w422]
              tunnel: [w414 w423] -> w406
              tunnel: w405 -> [w412 w424]
              tunnel: w402 -> [w411 _]
              tunnel: w401 -> [w413 _]
              frame False {
                n160 = case shown="True" w411 {
                  tunnel: [w415 w418] -> w414
                  tunnel: w413 -> [_ w417]
                  tunnel: w412 -> [w415 w416]
                  frame False {
                  }
                  frame True {
                    n161 = call <vilib>:"NodetoID.vi"("error in"=w416, "node ref"=w417) -> ("error out"=w420:errorcluster, "ID"=w421:string)  [unwired: 8 in]
                    n162 = call <vilib>:"Send Local Message.vi"("message name"="NodeDataChange", "message value"=w421, "error in"=w420) -> ("error out"=w418:errorcluster)  [unwired: 10 in, 2 out]
                  }
                }
              }
              frame True {
                n163 = call <vilib>:"NISE_error generator.vi"("error in"=w424, "source"="configuration tool main.vi", "append error message"=w422, "error code (0)"=538506) -> ("error out"=w423:errorcluster)  [unwired: 5 in]
              }
            }
          }
          frame True {
          }
        }
      }
      frame "RefreshNode" {
        # "Refreshes the node in the Tree, Sets the save flag to true. This case can be called from the UIs of the nodes"
        n164 = Unbundle By Name(w438) -> ("glyph manager"=w437:T9)
        n165 = call <vilib>:"IDtoNode.vi"("error in"=w445, "ID"=w443) -> ("error out"=w444:errorcluster, "invalid Id"=w441:bool, "node ref"=w442:T2)  [unwired: 7 in]
        n166 = case shown="False" w441 {
          tunnel: [w457 w460] -> w447
          tunnel: w444 -> [w453 w460]
          tunnel: w442 -> [w452 _]
          tunnel: w440 -> [w451 _]
          tunnel: [w450 w459] -> w439
          tunnel: w437 -> [w448 w459]
          frame False {
            n167 = call <vilib>:"SummaryWithGlyphManager.vi"("error in"=w453, "glyph manager"=w448, "node self ref"=w452) -> ("error out"=w455:errorcluster, "glyph manager out"=w449:T9, "summary"=w454:T18[])  [unwired: 6 in]
            n168 = call <vilib>:"RefreshSubTreeWithGlyphManager.vi"("error in"=w455, "glyph manager"=w449, "node information"=w454, "tree ref in"=w451) -> ("error out"=w458:errorcluster, "glyph manager out"=w450:T9, "tree ref out"=w456:refnum<vi>)  [unwired: 5 in]
            n169 = Close Reference(reference=w456, error in (no error)=w458) -> (error out=w457:errorcluster)
          }
          frame True {
          }
        }
        n170 = Bundle By Name(cluster=w438, "glyph manager"=w439) -> (w446:T1)
      }
      frame "RemoveNode" {
        n171 = call <vilib>:"IDtoNode.vi"("error in"=w466, "ID"=w467) -> ("error out"=w465:errorcluster, "invalid Id"=w462:bool, "node ref"=w464:T2)  [unwired: 7 in]
        n172 = case shown="False" w462 {
          tunnel: w465 -> [w474 w475]
          tunnel: w464 -> [w473 _]
          tunnel: [w470 w475] -> w463
          tunnel: w461 -> [w469 _]
          frame False {
            n173 = call <vilib>:"RemoveNode.vi"("error in"=w474, "node"=w473) -> ("error out"=w471:errorcluster, "node ID"=w472:string)  [unwired: 8 in]
            n174 = call <vilib>:"ClearTreeNode.vi"("error in"=w471, "tag"=w472, "tree reference"=w469) -> ("error out"=w470:errorcluster)  [unwired: 8 in]
          }
          frame True {
          }
        }
      }
      frame "PopulateTree" {
        n175 = Unbundle By Name(w498) -> ("standard events"=w490:T3, "glyph manager"=w487:T9, "root"=w494:T2)
        n176 = String Length(string=w479) -> (length=w478:i32)
        n177 = Greater Than 0?(x=w478) -> (x > 0?=w477:bool)
        n178 = call <vilib>:"SummaryWithGlyphManager.vi"("error in"=w496, "glyph manager"=w487, "depth"=0 ("Depth"), "node self ref"=w494) -> ("error out"=w495:errorcluster, "glyph manager out"=w486:T9, "summary"=w482:T18[])  [unwired: 5 in]
        n179 = Index Array(array=w482) -> (element=w481:T18)  [unwired: 1 in]
        n180 = control-ref of="This VI"() -> (w497:refnum<vi>)
        n181 = Unbundle By Name(w481) -> ("ID"=w480:string)
        n182 = call <vilib>:"RefreshEntireTreeWithGlyphManager.vi"("calling VI in"=w497, "error in"=w495, "glyph manager"=w486, "array"=w482, "tree ref in"=w485) -> ("error out"=w491:errorcluster, "glyph manager out"=w488:T9)  [unwired: 5 in]
        n183 = control-ref of="Sub Panel"() -> (w492:refnum<vi>)
        n184 = call <vilib>:"ClearSubPanelStandardEvents.vi"("error in"=w491, "standard events"=w490, "sub panel ref in"=w492) -> ("error out"=w484:errorcluster)  [unwired: 7 in, 1 out]
        n185 = Bundle By Name(cluster=w498, "glyph manager"=w488) -> (w489:T1)
        n186 = disable-structure shown="Enabled" {
          disable-tunnel: w485 -> [w501 w505]
          disable-tunnel: w484 -> [w500 w507]
          disable-tunnel: [w499 w506] -> w483
          disable-tunnel: w480 -> [_ w504]
          disable-tunnel: w477 -> [_ w503]
          frame Disabled {
            # "#Change - Condense tree"
            n187 = invoke class="Tree (strict)" method="Open/Close.Open/Close All"(reference=w501, error in=w500, "Open"=FALSE ("Open?")) -> (error out=w499:errorcluster)  [unwired: 1 in, 3 out]
          }
          frame Enabled {
            n188 = case shown="True" w503 {
              tunnel: w507 -> [w508 w512]
              tunnel: [w508 w511] -> w506
              tunnel: w505 -> [_ w510]
              tunnel: w504 -> [_ w509]
              frame False {
              }
              frame True {
                n189 = property class="Tree (strict)"(reference=w510, error in=w512, "Val(Sgnl)"=w509) -> (error out=w511:errorcluster)  [unwired: 1 out]
              }
            }
          }
        }
        n190 = local write "Status"("" ("Status")) -> ()
      }
      frame "CleansubPanel" {
        n191 = Unbundle By Name(w517) -> ("standard events"=w513:T3)
        n192 = control-ref of="Sub Panel"() -> (w519:refnum<vi>)
        n193 = call <vilib>:"ClearSubPanelStandardEvents.vi"("error in"=w518, "standard events"=w513, "sub panel ref in"=w519) -> ("error out"=w516:errorcluster, "sub panel ref out"=w515:refnum<vi>)  [unwired: 7 in]
        n194 = Close Reference(reference=w515, error in (no error)=w516) -> (error out=w514:errorcluster)
      }
      frame "ActivateNode" {
        n195 = Unbundle By Name(w522) -> ("standard events"=w521:T3)
        n196 = call <vilib>:"IDtoNode.vi"("error in"=w527, "ID"=w528) -> ("error out"=w520:errorcluster, "invalid Id"=w526:bool, "node ref"=w525:T2)  [unwired: 7 in]
        n197 = case shown="False" w526 {
          tunnel: w525 -> [w535 _]
          tunnel: [w536 w537] -> w524
          tunnel: w520 -> [w533 w537]
          tunnel: w523 -> [w531 _]
          tunnel: w521 -> [w529 _]
          frame False {
            n198 = control-ref of="Sub Panel"() -> (w532:refnum<vi>)
            n199 = call <vilib>:"ClearSubPanelStandardEvents.vi"("error in"=w533, "standard events"=w529, "sub panel ref in"=w532) -> ("error out"=w534:errorcluster, "sub panel ref out"=w530:refnum<vi>)  [unwired: 7 in]
            n200 = call <vilib>:"LoadNodeUIStandardEvents.vi"("user event out"=w529, "error in"=w534, "sub panel ref in"=w530, "main queue"=w531, "node"=w535) -> ("error out"=w536:errorcluster)  [unwired: 6 in]
          }
          frame True {
          }
        }
      }
      frame "Move" {
        n201 = Unflatten From String(type=T14 {"node ref"=refnum, "new parent"=refnum} ("Cluster"), binary string=w548, error in (no error)=w546) -> (value=w545:T14, error out=w544:errorcluster)  [unwired: 2 in, 1 out]
        n202 = Unbundle By Name(w545) -> ("node ref"=w539:T2, "new parent"=w538:T2)
        n203 = call <vilib>:"MoveNode.vi"("error in"=w544, "new parent"=w538, "node"=w539) -> ("error out"=w542:errorcluster)  [unwired: 8 in]
        n204 = call <vilib>:"Send Local Message.vi"("message queue in"=w540, "message name"="PopulateTree", "error in"=w542) -> ("error out"=w541:errorcluster)  [unwired: 10 in, 2 out]
      }
      frame "NodeDataChange" {
        n205 = call <vilib>:"Send Local Message.vi"("message queue in"=w553, "message name"="RefreshNode", "message value"=w555, "error in"=w556) -> ("error out"=w554:errorcluster)  [unwired: 9 in, 2 out]
        n206 = Bundle By Name(cluster=w557, "unsaved changes"=TRUE) -> (w551:T1)
      }
    }
  }
  n207 = while "User Interface Event Handler" {
    tunnel: w26 -> [w566]
    tunnel: w25 -> [w562]
    tunnel: w18 -> [w561]
    tunnel: [w560] -> w14
    shift-right: [w558] -> _
    shift-left: w11 -> [w559]
    stop <- w565 stop-if-true
    n208 = event shown="[3] \"VeriStand Version\": Value Change" {
      selector: w561 -> [_ _ _ _ _ _ _ _ _ _ _ _ _]
      dyn-events: [_ _ _ _ _ _ _ _ _ _ _ _ _] -> w560
      timeout: 1000 -> [_ _ _ _ _ _ _ _ _ _ _ _ _]
      tunnel: w566 -> [w570 w579 w604 w654 w661 w689 w718 w726 w756 w761 w772 w779 w826]
      tunnel: [_ _ _ _ _ _ TRUE _ _ _ _ _ _] -> w565
      tunnel: [w570 w579 w603 w654 w661 w687 w714 w726 w753 w761 w770 w778 w827] -> w564
      tunnel: [w569 w575 w602 _ w655 w686 w715 w722 w752 w758 w768 w776 _] -> w563
      tunnel: w562 -> [w569 w578 w601 _ w656 w688 w716 w725 w751 w760 w769 w777 _]
      tunnel: w559 -> [w568 w571 w597 w653 w657 w673 w713 w721 w750 w757 w767 w774 w824]
      tunnel: [w568 w571 w597 w653 w658 w673 w713 w721 w750 w757 w767 w774 w824] -> w558
      event Timeout {
        # "Timeout code can be added here for autosave or Lock Screen"
        n209 = event-data() -> ()  [unwired: 1 in, 1 out]
      }
      event "View": Shortcut Menu Activation? {
        n210 = event-data() -> ("CtlRef"=w585:refnum<vi>, "Coords"=w584:T19, "MenuRef"=w581:refnum<k9>)  [unwired: 1 in]
        n211 = invoke class="Tree (strict)" method="Point To Row Column"(reference=w585, error in=w578, "Point"=w584) -> (error out=w577:errorcluster, "Tag"=w583:string)  [unwired: 5 in, 6 out]
        n212 = call <vilib>:"IDtoNode.vi"("error in"=w577, "ID"=w583) -> ("error out"=w573:errorcluster, "invalid Id"=w580:bool, "node ref"=w582:T2)  [unwired: 7 in]
        n213 = case shown="False" w580 {
          tunnel: w582 -> [w590 _]
          tunnel: w581 -> [w589 _]
          tunnel: [w588 _] -> w576
          tunnel: [w587 _] -> w574
          tunnel: w573 -> [w586 w596]
          tunnel: [w586 w596] -> w572
          frame False {
            n214 = in-place {
              in-place-border: w589 -> [w593]
              in-place-border: [w591] -> w588
              n215 = in-place-dvr #8(w590) -> (w595:refnum<class "NISE_CEF_Node.lvclass">, w592:errorcluster)
              n216 = call-dynamic "ShortcutMenu.vi"("error in"=w592, "menu ref in"=w593, "node in"=w595) -> ("error out"=w591:errorcluster, "node out"=w594:refnum<class "NISE_CEF_Node.lvclass">)  [unwired: 6 in, 1 out]
              n217 = in-place-dvr #8(w594) -> (w587:errorcluster)  [unwired: 1 out]
            }
          }
          frame True {
          }
        }
        n218 = Merge Errors(w574, w576, w572) -> (w575:errorcluster)
        n219 = event-data() -> ()  [unwired: 2 in, 1 out]
      }
      event "View": Shortcut Menu Selection (User) {
        n220 = event-data() -> ("ItemPath"=w598:string, "CtlRef"=w607:refnum<vi>, "Coords"=w608:T19)  [unwired: 1 in]
        n221 = invoke class="Tree (strict)" method="Point To Row Column"(reference=w607, error in=w601, "Point"=w608) -> (error out=w600:errorcluster, "Tag"=w599:string)  [unwired: 5 in, 6 out]
        n222 = Match Pattern(string=w598, regular expression=":") -> (before substring=w606:string, after substring=w605:string)  [unwired: 1 in, 2 out]
        n223 = case shown="\"Add\"" w606 {
          selector: w606 -> [w610 _ _ _ _]
          tunnel: w605 -> [_ _ _ w634 w638]
          tunnel: w604 -> [w617 w624 w630 w636 w645]
          tunnel: w599 -> [w612 w622 w628 w633 w644]
          tunnel: [w614 w621 w627 w632 w642] -> w603
          tunnel: [w615 w620 w625 w631 w640] -> w602
          tunnel: w600 -> [w616 w619 w626 w635 w641]
          frame Default {
            n224 = Concatenate Strings(w610, ":" ("string"), w612) -> (w613:string)
            n225 = call <vilib>:"Send Local Message.vi"("message queue in"=w617, "message name"="CustomMenuAction" ("Message Name"), "message value"=w613, "error in"=w616) -> ("message queue out"=w614:T12, "error out"=w615:errorcluster)  [unwired: 9 in, 1 out]
          }
          frame "Remove" {
            n226 = call <vilib>:"Send Local Message.vi"("message queue in"=w624, "message name"="RemoveNode" ("Message Name"), "message value"=w622, "error in"=w619) -> ("message queue out"=w621:T12, "error out"=w620:errorcluster)  [unwired: 9 in, 1 out]
          }
          frame "Duplicate" {
            n227 = call <vilib>:"Send Local Message.vi"("message queue in"=w630, "message name"="Duplicate" ("Message Name"), "message value"=w628, "error in"=w626) -> ("message queue out"=w627:T12, "error out"=w625:errorcluster)  [unwired: 9 in, 1 out]
          }
          frame "Add" {
            n228 = call "Send Message to Create Child Object.vi"("Error In"=w635, "ID of Node to Add To"=w633, "node type"=w634, "Queue in"=w636) -> ("Error Out"=w631:errorcluster, "Queue Out"=w632:T12)  [unwired: 6 in]
          }
          frame "New" {
            n229 = Match Pattern(string=w638, regular expression=":") -> (after substring=w637:string)  [unwired: 1 in, 3 out]
            n230 = Bundle By Name(cluster=T13 {"node type"="", "to add to"=""} ("input cluster"), "node type"=w637, "to add to"=w644) -> (w646:T13)
            n231 = Flatten To String(anything=w646) -> (data string=w647:string)  [unwired: 3 in, 2 out]
            n232 = call <vilib>:"Send Local Message.vi"("message queue in"=w645, "message name"="AddNode" ("Message Name"), "message value"=w647, "error in"=w641) -> ("message queue out"=w642:T12, "error out"=w640:errorcluster)  [unwired: 9 in, 1 out]
          }
        }
      }
      event "VeriStand Version": Value Change {
        n233 = event-data() -> ("NewVal"=w650:string)  [unwired: 1 in, 5 out]
        n234 = control-ref of="This VI"() -> (w649:refnum<vi>)
        n235 = global write "Global Settings.vi" "VeriStand Version (String)"(w650) -> ()
        n236 = property class="VI"(reference=w649) -> ("Panel"=w652:refnum<vi>)  [unwired: 1 in, 2 out]
        n237 = property class="Pnl"(reference=w652, "DeferPanUpdts"=FALSE ("Defer Panel Updates")) -> ()  [unwired: 1 in, 2 out]
      }
      event "Target Project": Value Change {
        n238 = event-data() -> ("OldVal"=w659:string)  [unwired: 1 in, 5 out]
        n239 = case shown="Default" "Target Project" {
          selector: "Target Project" -> [_ w671]
          tunnel: w659 -> [w666 _]
          tunnel: [w664 w670] -> w658
          tunnel: w657 -> [_ w670]
          tunnel: w656 -> [w663 w669]
          tunnel: [w662 w668] -> w655
          frame "Refresh..." {
            n240 = control-ref of="Target Project"() -> (w667:refnum<vi>)
            n241 = call "Initialize Target Project.vi"("error in (no error)"=w663, "ComboBox in"=w667) -> ("error out"=w665:errorcluster, "Projects"=w664:T11)  [unwired: 8 in]
            n242 = call "Set Target Project.vi"("error in (no error)"=w665, "Target Project"=w666, "Projects"=w664, "ComboBox Ref"=w667) -> ("error out"=w662:errorcluster)  [unwired: 7 in]
          }
          frame Default {
            n243 = control-ref of="Target Project"() -> (w672:refnum<vi>)
            n244 = call "Set Target Project.vi"("error in (no error)"=w669, "Target Project"=w671, "Projects"=w670, "ComboBox Ref"=w672) -> ("error out"=w668:errorcluster)  [unwired: 7 in]
          }
        }
      }
      event "View": Drop {
        n245 = event-data() -> ("CtlRef"=w692:refnum<vi>, "Coords"=w691:T19)  [unwired: 1 in]
        n246 = invoke class="Tree (strict)" method="Point To Row Column"(reference=w692, error in=w688, "Point"=w691) -> (reference out=w690:refnum<vi>, error out=w685:errorcluster, "Tag"=w682:string)  [unwired: 5 in, 5 out]
        n247 = call <vilib>:"ValidDragDrop.vi"("error in"=w685, "drag over"=w682, "Tree Ref in"=w690) -> ("Error Out"=w677:errorcluster, "Accepted"=w680:bool, "Drag"=w684:string, "Tree Ref out"=w694:refnum<vi>)  [unwired: 1 in, 4 out]
        n248 = call <vilib>:"IDtoNode.vi"("error in"=w677, "ID"=w682) -> ("error out"=w678:errorcluster, "invalid Id"=w675:bool, "node ref"=w681:T2)  [unwired: 7 in]
        n249 = call <vilib>:"IDtoNode.vi"("error in"=w678, "ID"=w684) -> ("error out"=w676:errorcluster, "invalid Id"=w674:bool, "node ref"=w683:T2)  [unwired: 7 in]
        n250 = Compound Arithmetic op=AND(w680, invert w675, invert w674) -> (w679:bool)
        n251 = case shown="True" w679 {
          tunnel: w684 -> [_ w710]
          tunnel: w694 -> [_ w712]
          tunnel: [_ TRUE] -> w693
          tunnel: w682 -> [_ w708]
          tunnel: w689 -> [w696 w707]
          tunnel: [w696 w703] -> w687
          tunnel: [w695 w702] -> w686
          tunnel: w683 -> [_ w698]
          tunnel: w681 -> [_ w697]
          tunnel: w676 -> [w695 w699]
          frame False {
          }
          frame True {
            n252 = invoke class="Tree (strict)" method="Edit Tree Items.Move Item"(reference=w712, error in=w699, "tag"=w710, "New Parent"=w708) -> (error out=w700:errorcluster)  [unwired: 3 in, 6 out]
            n253 = Bundle By Name(cluster=T14 {"node ref"=refnum, "new parent"=refnum} ("Cluster"), "new parent"=w697, "node ref"=w698) -> (w706:T14)
            n254 = Flatten To String(anything=w706, error in (no error)=w700) -> (data string=w705:string, error out=w701:errorcluster)  [unwired: 2 in, 1 out]
            n255 = call <vilib>:"Send Local Message.vi"("message queue in"=w707, "message name"="Move", "message value"=w705, "error in"=w701) -> ("message queue out"=w703:T12, "error out"=w702:errorcluster)  [unwired: 9 in, 1 out]
          }
        }
        n256 = event-data("Accepted?"=w693) -> ()  [unwired: 1 in, 1 out]
      }
      event "Exit": Value Change {
        # "Exit the application                                           >> Stop this message generator loop    Cleaning errors if the other loop stop this one"
        n257 = event-data() -> ()  [unwired: 1 in, 1 out]
        n258 = call <vilib>:"Send Local Message.vi"("message queue in"=w718, "message name"="Close", "error in"=w716) -> ("message queue out"=w714:T12, "error out"=w719:errorcluster)  [unwired: 10 in, 1 out]
        n259 = call <vilib>:"Clear Errors.vi"("error in (no error)"=w719) -> ("error out"=w715:errorcluster)  [unwired: 5 in, 1 out]
      }
      event "View": Drag Starting? {
        n260 = event-data() -> ("Data"=w732:T20, "CtlRef"=w734:refnum<vi>, "Coords"=w733:T19)  [unwired: 1 in]
        n261 = invoke class="Tree (strict)" method="Point To Row Column"(reference=w734, error in=w725, "Point"=w733) -> (error out=w724:errorcluster, "Tag"=w731:string)  [unwired: 5 in, 6 out]
        n262 = call <vilib>:"IDtoNode.vi"("error in"=w724, "ID"=w731) -> ("error out"=w723:errorcluster, "invalid Id"=w730:bool, "node ref"=w729:T2)  [unwired: 7 in]
        n263 = case shown="False" w730 {
          tunnel: w729 -> [w742 _]
          tunnel: [w739 TRUE ("Removable")] -> w727
          tunnel: w723 -> [w738 w748]
          tunnel: [w735 w748] -> w722
          frame False {
            n264 = in-place {
              in-place-border: [w745] -> w741
              in-place-border: w738 -> [w744]
              in-place-border: [w743] -> w737
              n265 = in-place-dvr #9(w742) -> (w747:refnum<class "NISE_CEF_Node.lvclass">)  [unwired: 1 out]
              n266 = call-dynamic "EditOptions.vi"("error in"=w744, "node in"=w747) -> ("error out"=w743:errorcluster, "edit options"=w745:T21, "node out"=w746:refnum<class "NISE_CEF_Node.lvclass">)  [unwired: 6 in, 1 out]
              n267 = in-place-dvr #9(w746) -> (w736:errorcluster)  [unwired: 1 out]
            }
            n268 = Unbundle By Name(w741) -> ("movable"=w740:bool)
            n269 = Merge Errors(w736, w737) -> (w735:errorcluster)
            n270 = Not(x=w740) -> (.not. x?=w739:bool)
          }
          frame True {
          }
        }
        n271 = event-data("Data"=w732, "Drag Mode"=enum32{"copy or move", "copy only", "move only"}."move only", "Discard?"=w727) -> ()  [unwired: 1 in, 1 out]
      }
      event "View": Value Change {
        n272 = event-data() -> ("NewVal"=w754:string)  [unwired: 1 in]
        n273 = call <vilib>:"Send Local Message.vi"("message queue in"=w756, "message name"="ActivateNode" ("Message Name"), "message value"=w754, "error in"=w751) -> ("message queue out"=w753:T12, "error out"=w752:errorcluster)  [unwired: 9 in, 1 out]
      }
      event "View": event type 3.0.xa000003a {
        n274 = event-data() -> ("CtlRef"=w766:refnum<vi>, "Coords"=w763:T19)  [unwired: 1 in]
        n275 = invoke class="Tree (strict)" method="Point To Row Column"(reference=w766, error in=w760, "Point"=w763) -> (reference out=w765:refnum<vi>, error out=w759:errorcluster, "Tag"=w764:string)  [unwired: 5 in, 5 out]
        n276 = call <vilib>:"ValidDragDrop.vi"("error in"=w759, "drag over"=w764, "Tree Ref in"=w765) -> ("Error Out"=w758:errorcluster, "Accepted"=w762:bool)  [unwired: 1 in, 6 out]
        n277 = event-data("Accepted?"=w762) -> ()  [unwired: 1 in, 1 out]
      }
      event Panel Close? {
        # "Intercepts the upper right close panel operation to allow a smooth shutdown as opposed to immediately killing the app."
        n278 = event-data() -> ()  [unwired: 1 in, 1 out]
        n279 = call <vilib>:"Send Local Message.vi"("message queue in"=w772, "message name"="Close?", "error in"=w769) -> ("message queue out"=w770:T12, "error out"=w768:errorcluster)  [unwired: 10 in, 1 out]
        n280 = event-data("Discard?"=TRUE) -> ()  [unwired: 1 in, 1 out]
      }
      event Menu Selection (User) {
        # "#USERCFG It is needed to add a Case for Every item on the menu"
        n281 = event-data() -> ("ItemTag"=w775:string, "ItemPath"=w780:string)  [unwired: 1 in]
        n282 = case shown="Default" w780 {
          selector: w780 -> [w784 _ _ _ _ _ _]
          tunnel: w779 -> [w789 w794 w799 w804 w809 w814 w823]
          tunnel: [w789 w790 w795 w800 w805 w810 w820] -> w778
          tunnel: w777 -> [w786 w792 w797 w802 w807 w812 w819]
          tunnel: [w785 w791 w796 w801 w806 w811 w817] -> w776
          tunnel: w775 -> [w783 _ _ _ _ _ _]
          frame Default {
            n283 = Concatenate Strings(w783, "::" ("string"), w784) -> (w782:string)
            n284 = call <vilib>:"NISE_error generator.vi"("error in"=w786, "source"="configuration tool main.vi", "append error message"=w782, "error code (0)"=538506) -> ("error out"=w785:errorcluster)  [unwired: 5 in]
          }
          frame "_File:_New" {
            n285 = call <vilib>:"Send Local Message.vi"("message queue in"=w794, "message name"="New?" ("Message Name"), "error in"=w792) -> ("message queue out"=w790:T12, "error out"=w791:errorcluster)  [unwired: 10 in, 1 out]
          }
          frame "_File:_Open" {
            n286 = call <vilib>:"Send Local Message.vi"("message queue in"=w799, "message name"="Open?" ("Message Name"), "error in"=w797) -> ("message queue out"=w795:T12, "error out"=w796:errorcluster)  [unwired: 10 in, 1 out]
          }
          frame "_File:_Save" {
            n287 = call <vilib>:"Send Local Message.vi"("message queue in"=w804, "message name"="Save" ("Message Name"), "error in"=w802) -> ("message queue out"=w800:T12, "error out"=w801:errorcluster)  [unwired: 10 in, 1 out]
          }
          frame "_File:Save As..." {
            n288 = call <vilib>:"Send Local Message.vi"("message queue in"=w809, "message name"="SaveAs" ("Message Name"), "error in"=w807) -> ("message queue out"=w805:T12, "error out"=w806:errorcluster)  [unwired: 10 in, 1 out]
          }
          frame "_File:_Exit" {
            n289 = call <vilib>:"Send Local Message.vi"("message queue in"=w814, "message name"="Close?" ("Message Name"), "error in"=w812) -> ("message queue out"=w810:T12, "error out"=w811:errorcluster)  [unwired: 10 in, 1 out]
          }
          frame "_Tools:Multiple Parameter Editor" {
            n290 = call <vilib>:"Send Local Message.vi"("message queue in"=w823, "message name"="CleansubPanel", "error in"=w819) -> ("message queue out"=w822:T12, "error out"=w818:errorcluster)  [unwired: 10 in, 1 out]
            n291 = call <vilib>:"Send Local Message.vi"("message queue in"=w822, "message name"="Custom View" ("Message Name"), "message value"="Multiple Variable Editor" ("Message Name"), "error in"=w818) -> ("message queue out"=w820:T12, "error out"=w817:errorcluster)  [unwired: 9 in, 1 out]
          }
        }
      }
      event User Event {
        n292 = event-data() -> ("node ref"=w825:T2)  [unwired: 1 in]
        n293 = call <vilib>:"NodetoID.vi"("node ref"=w825) -> ("ID"=w828:string)  [unwired: 9 in, 1 out]
        n294 = call <vilib>:"Send Local Message.vi"("message queue in"=w826, "message name"="NodeDataChange", "message value"=w828) -> ("message queue out"=w827:T12)  [unwired: 10 in, 2 out]
      }
    }
    n295 = call "Error.vi"("error in (no error)"=w563, "message queue in"=w564) -> ()  [unwired: 9 in, 1 out]
  }
  n296 = Unregister For Events(event registration refnum=w14) -> (error out=w15:errorcluster)  [unwired: 1 in]
  n297 = Merge Errors(w15, w20) -> (w16:errorcluster)
  n298 = call <vilib>:"DestroyStandardEvents.vi"("error in"=w16, "standard events"=w19) -> ("error out"=w6:errorcluster)  [unwired: 9 in]
  n299 = invoke class="VI" method="Save.Instrument"(error in=w6) -> (reference out=w5:refnum<vi>, error out=w4:errorcluster)  [unwired: 5 in, 4 out]
  n300 = disable-structure shown="Disabled" {
    disable-tunnel: w5 -> [w831 _]
    disable-tunnel: w4 -> [w830 _]
    frame Disabled {
      n301 = invoke class="VI" method="FP.Close"(reference=w831, error in=w830) -> ()  [unwired: 1 in, 3 out]
    }
    frame Enabled {
    }
  }
  "Status" <- "No configuration loaded" ("Status")
